vi "automatic_wait.vi"(7 "transition_queue":refnum<queue>, 8 "error in (no error)":errorcluster, 10 "data":variant, 11 "recipe_data":variant) -> (0 "error out":errorcluster)   [LabVIEW 2015, in "lv-recipe-machine.lvlib" / "example_01.lvlib"]
doc: "automatic_wait.vi executes similarly to the manual_wait.vi with the exception that it can be stopped mid-run using the fg_stop.vi. IT will wait the configured amount o time and output amount of time elapsed."
uses:
  example_01.lvlib
  public/_controls/transition.ctl
  _controls/steps_actions_data.ctl
  _controls/steps_actions.ctl
  lv-recipe-machine.lvlib
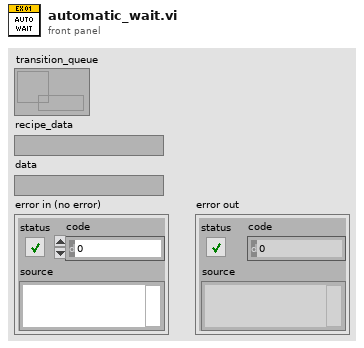
[diagram p1: front panel]
types:
  T1 = typedef "lv-recipe-machine.lvlib/example_01.lvlib/steps_actions.ctl" = enum16{"<steps_actions>", "manual_random", "manual_comparison", "manual_wait", "auto_random", "auto_wait", "criteria_initialize", "criteria_count", "criteria_comparison", "transition_simple", "transition_count", "transition_comparison", "launch_wait", "<null>"}
  T2 = typedef "lv-recipe-machine.lvlib/example_01.lvlib/steps_actions_data.ctl" = cluster{"step_action":T1, "data":variant}
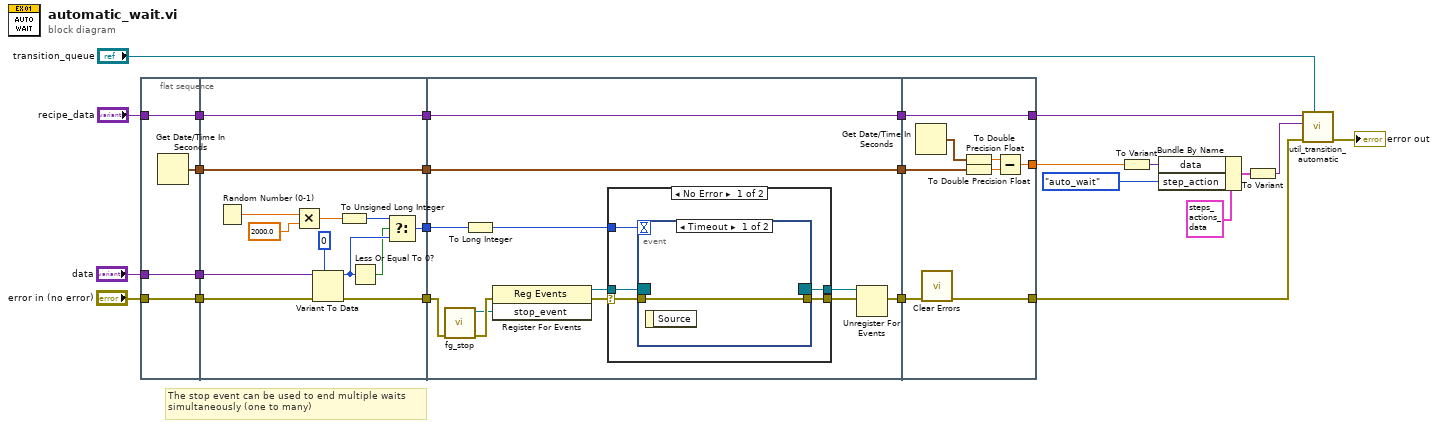
[diagram p0: block diagram]
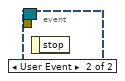
[diagram p2: hidden frame]
diagram:
  # "The stop event can be used to end multiple waits\nsimultaneously (one to many)"
  n1 = flat-sequence {
    tunnel: "data" -> [w28]
    tunnel: "error in (no error)" -> [w27]
    tunnel: [w28] -> w24
    tunnel: [w27] -> w23
    tunnel: [w26] -> w22
    tunnel: "recipe_data" -> [w25]
    tunnel: [w25] -> w6
    tunnel: w24 -> [w34]
    tunnel: w23 -> [w35]
    tunnel: w22 -> [w41]
    tunnel: [w41] -> w21
    tunnel: [w33] -> w20
    tunnel: [w30] -> w19
    tunnel: w6 -> [w29]
    tunnel: [w29] -> w4
    tunnel: w21 -> [w51]
    tunnel: [w51] -> w18
    tunnel: w20 -> [w50]
    tunnel: w19 -> [w47]
    tunnel: [w46] -> w9
    tunnel: [w42] -> w5
    tunnel: w4 -> [w42]
    tunnel: w18 -> [w62]
    tunnel: [w67] -> w16
    tunnel: [w66] -> w10
    tunnel: w9 -> [w65]
    tunnel: [w64] -> w3
    tunnel: w5 -> [w64]
    frame #0 {
      n2 = Get Date/Time In Seconds() -> (seconds since 1Jan1904=w26:timestamp)
    }
    frame #1 {
      n3 = Random Number (0-1)() -> (number: 0 to 1=w37:dbl)
      n4 = Multiply(x=w37, y=2000.0) -> (x*y=w39:dbl)
      n5 = Variant To Data(error in=w35, type=u32 0, Variant=w34) -> (data=w32:u32, error out=w30:errorcluster)
      n6 = To Unsigned Long Integer(number=w39) -> (unsigned 32bit integer=w40:u32)
      n7 = Less Or Equal To 0?(x=w32) -> (x <= 0?=w31:bool)
      n8 = Select(t=w40, s=w31, f=w32) -> (s? t:f=w33:u32)
    }
    frame #2 {
      n9 = call "fg_stop.vi"("error in (no error)"=w47) -> ("error out"=w52:errorcluster, "stop_event"=w48:refnum<user-event>)  [unwired: 9 in]
      n10 = To Long Integer(number=w50) -> (32bit integer=w49:i32)
      n11 = register-events(error in=w52, w48) -> (reference out=w44:refnum<event-registration>, error out=w45:errorcluster)  [unwired: 1 in]
      n12 = case shown="No Error" w45 {
        selector: w45 -> [w55 w59]
        tunnel: w49 -> [w57 _]
        tunnel: [w56 w59] -> w46
        tunnel: w44 -> [w54 w60]
        tunnel: [w53 w60] -> w43
        frame No Error {
          n13 = event shown="[0] Timeout" {
            selector: w54 -> [_ _]
            dyn-events: [_ _] -> w53
            timeout: w57 -> [_ _]
            tunnel: [w58 _] -> w56
            tunnel: w55 -> [w58 _]
            event Timeout {
              n14 = event-data() -> ()  [unwired: 1 in, 1 out]
            }
            event User Event {
              n15 = event-data() -> ()  [unwired: 1 in, 1 out]
            }
          }
        }
        frame Error {
        }
      }
      n16 = Unregister For Events(event registration refnum=w43) -> ()  [unwired: 1 in, 1 out]
    }
    frame #3 {
      n17 = Get Date/Time In Seconds() -> (seconds since 1Jan1904=w68:timestamp)
      n18 = call <vilib>:"Clear Errors.vi"("error in (no error)"=w65) -> ("error out"=w66:errorcluster)  [unwired: 5 in, 1 out]
      n19 = To Double Precision Float(number=w68) -> (double precision float=w63:dbl)
      n20 = To Double Precision Float(number=w62) -> (double precision float=w61:dbl)
      n21 = Subtract(x=w63, y=w61) -> (x-y=w67:dbl)
    }
  }
  n22 = To Variant(anything=w16) -> (Variant=w17:variant)
  n23 = Bundle By Name(cluster=T2 {"step_action"=enum."<steps_actions>", "data"=variant}, "data"=w17, "step_action"=steps_actions."auto_wait" ("automatic_steps")) -> (w14:T2)
  n24 = To Variant(anything=w14) -> (Variant=w8:variant)
  n25 = call "util_transition_automatic.vi"("transition_queue"="transition_queue", "error in (no error)"=w10, "data"=w8, "recipe_data"=w3) -> ("error out"=→"error out":errorcluster)  [unwired: 7 in]
